vi "RT Error Handler - UI Commands.vi"(8 "error in (no error)":errorcluster, 11 "Message Queue":refnum<queue>) -> (3 "dup Message Queue":refnum<queue>)   [LabVIEW 2018]
uses:
  Support/Message Queue/Message Cluster.ctl
  Support/Message Queue/Message.ctl
  support/Message Queue/Message Queue.lvlib
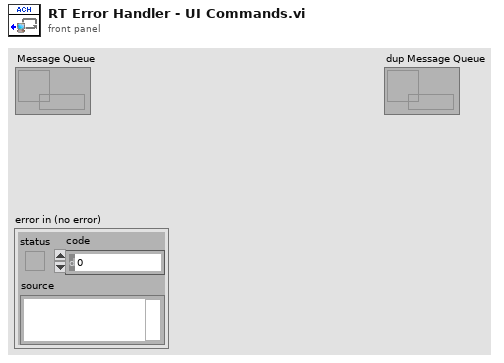
[diagram p1: front panel]
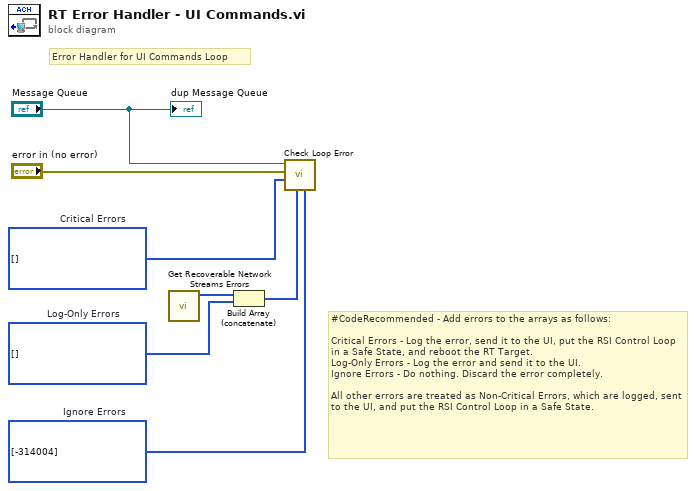
[diagram p0: block diagram]
diagram:
  w6 = i32[] [-314004]  # Ignore Errors
  w2 = i32[] []  # Log-Only Errors
  w7 = i32[] []  # Critical Errors
  # "#CodeRecommended - Add errors to the arrays as follows:\n\nCritical Errors - Log the error, send it to the UI, put the RSI Control Loop in a Safe State, and reboot the RT Target.\nLog-Only Errors - Log the error and send it to the UI.\nIgnore Errors - Do nothing. Discard the error completely.\n\nAll other errors are treated as Non-Critical Errors, which are logged, sent to the UI, and put the RSI Control Loop in a Safe State."
  # "Error Handler for UI Commands Loop"
  n1 = call "Get Recoverable Network Streams Errors.vi"() -> ("recoverable network streams errors"=w3:i32[])  [unwired: 11 in]
  n2 = Build Array (concatenate)(w3, w2) -> (w1:i32[])
  n3 = call "Check Loop Error.vi"("Ignore Errors"=w6, "Log-Only Errors"=w1, "Critical Errors"=w7, "error to process"="error in (no error)", "Message Queue"="Message Queue") -> ()  [unwired: 5 in, 2 out]
  "dup Message Queue" <- "Message Queue"
